vi "New Parameterized Test Case.vi"(8 "error in (no error)":errorcluster) -> (0 "error out":errorcluster)   [LabVIEW 2020]
uses:
  <vilib>/Utility/error.llb/Error Cluster From Error Code.vi
  <vilib>/ErrorRing/Error Ring.xnode
panel:
  in  "Debug?":bool
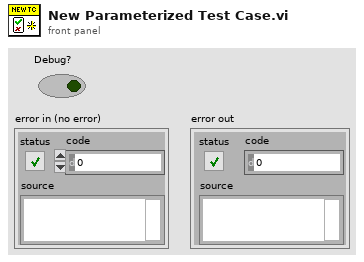
[diagram p1: front panel]
types:
  T1 = enum32{"Invalid", "Standard", "Closed", "Hidden", "Minimized", "Maximized"}
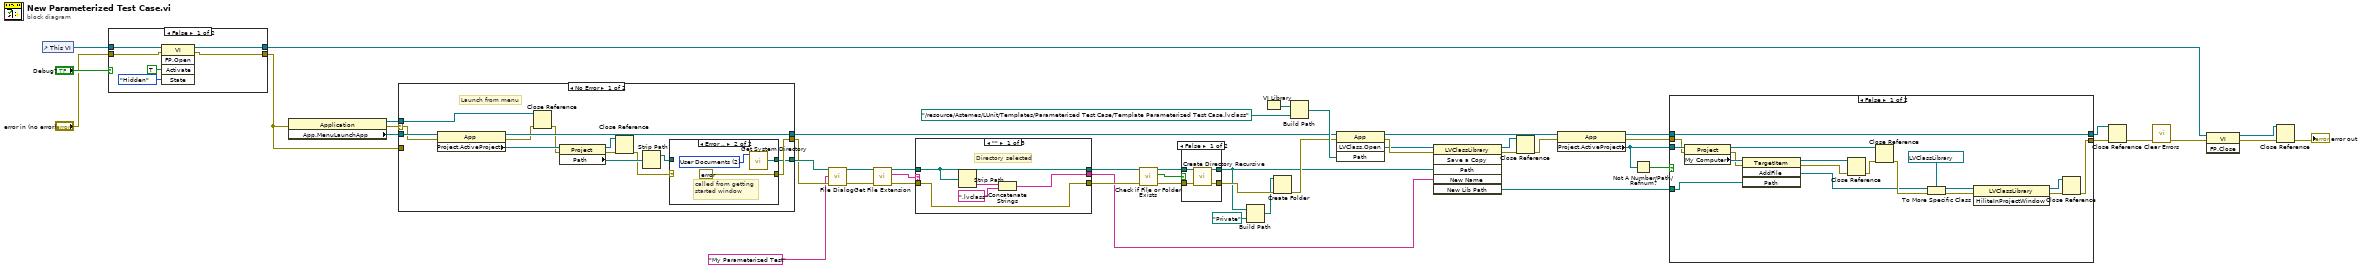
[diagram p0: block diagram]
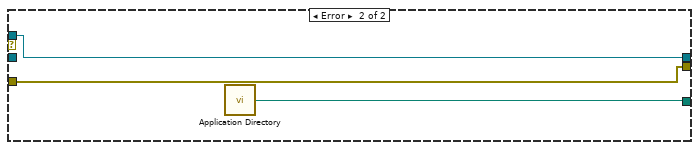
[diagram p3: hidden frame]
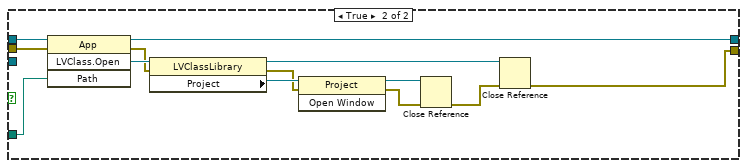
[diagram p5: hidden frame]
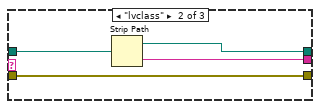
[diagram p6: hidden frame]
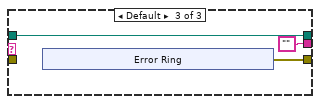
[diagram p7: hidden frame]
diagram:
  n1 = control-ref of="This VI"() -> (w21:refnum<vi>)
  n2 = case shown="False" "Debug?" {
    tunnel: w21 -> [w55 w57]
    tunnel: [w54 w57] -> w19
    tunnel: "error in (no error)" -> [w51 w56]
    tunnel: [w50 w56] -> w10
    frame False {
      n3 = invoke class="VI" method="FP.Open"(reference=w55, error in=w51, "Activate"=TRUE ("Activate?"), "State"=T1."Hidden") -> (reference out=w54:refnum<vi>, error out=w50:errorcluster)  [unwired: 1 in, 3 out]
    }
    frame True {
    }
  }
  n4 = property class="Application"(error in=w10) -> (reference out=w16:refnum<vi>, error out=w24:errorcluster, "App.MenuLaunchApp"=w49:refnum<vi>)  [unwired: 1 in]
  n5 = case shown="No Error" w24 {
    selector: w24 -> [w66 _]
    tunnel: [w69 w79] -> w12
    tunnel: w49 -> [w67 _]
    tunnel: [w60 w78] -> w8
    tunnel: w10 -> [_ w78]
    tunnel: w16 -> [w71 w79]
    tunnel: [w59 w77] -> w9
    frame No Error {
      # "Launch from menu"
      n6 = property class="App"(reference=w67, error in=w66) -> (reference out=w69:refnum<vi>, error out=w68:errorcluster, "Project.ActiveProject"=w70:refnum<vi>)
      n7 = Close Reference(reference=w71, error in (no error)=w68) -> (error out=w65:errorcluster)
      n8 = property class="Project"(reference=w70, error in=w65) -> (reference out=w63:refnum<vi>, error out=w64:errorcluster, "Path"=w62:path)
      n9 = Close Reference(reference=w63, error in (no error)=w64) -> (error out=w61:errorcluster)
      n10 = Strip Path(path=w62) -> (stripped path=w58:path)  [unwired: 1 out]
      n11 = case shown="Error .." w61 {
        selector: w61 -> [w73 _]
        tunnel: [w73 errorcluster {"status"=FALSE, "code"=0, "source"=""} ("error IO")] -> w60
        tunnel: [w72 w74] -> w59
        tunnel: w58 -> [w72 _]
        frame No Error {
        }
        frame Error {
          w75 = 2 items=["User Home"=0, "User Desktop"=1, "User Documents"=2, "User Application Data"=3, "User Preferences"=4, "User Temporary"=5, "Public Documents"=6, "Public Application Data"=7, "Public Preferences"=8, "Public Cache"=13, "System Core Libraries"=9, "System Installed Libraries"=10, "Application Files"=11, "Boot Volume Root"=12] ("system directory type")
          # "called from getting started window"
          n12 = call <vilib>:"Get System Directory.vi"("system directory type"=w75) -> ("system directory"=w74:path)  [unwired: 10 in]
        }
      }
    }
    frame Error {
      n13 = call <vilib>:"Application Directory.vi"() -> ("Application Directory"=w77:path)
    }
  }
  n14 = call "File Dialog"("start path"=w9, "default name"="My Parameterized Test", "error in"=w8) -> ("selected path"=w45:path, "error out"=w7:errorcluster)  [unwired: 9 in, 2 out]
  n15 = call <vilib>:"Get File Extension.vi"("error in (no error)"=w7, "file"=w45) -> ("error out"=w48:errorcluster, "lowercase file extension"=w47:string, "dup file"=w46:path)  [unwired: 5 in, 2 out]
  n16 = case shown="\"\"" w47 {
    tunnel: w48 -> [w80 w85 _]
    tunnel: w46 -> [w81 w88 w89]
    tunnel: [w80 w85 w91] -> w43
    tunnel: [w82 w87 "" ("name")] -> w39
    tunnel: [w81 w86 w89] -> w44
    frame "" {
      # "Directory selected"
      n17 = Strip Path(path=w81) -> (name=w84:string)  [unwired: 1 out]
      n18 = Concatenate Strings(w84, ".lvclass" ("string")) -> (w82:string)
    }
    frame "lvclass" {
      n19 = Strip Path(path=w88) -> (stripped path=w86:path, name=w87:string)
    }
    frame Default {
      n20 = xnode "Error Ring"() -> ("error out"=w91:errorcluster)
    }
  }
  n21 = call <vilib>:"Check if File or Folder Exists.vi"("error in (no error)"=w43, "path"=w44) -> ("error out"=w42:errorcluster, "file or folder exists?"=w40:bool, "dup path"=w41:path)  [unwired: 7 in]
  n22 = case shown="False" w40 {
    tunnel: w42 -> [w99 w100]
    tunnel: w41 -> [w98 w101]
    tunnel: [w97 w101] -> w3
    tunnel: [w96 w100] -> w6
    frame False {
      n23 = call <vilib>:"Create Directory Recursive.vi"("error in (no error)"=w99, "directory"=w98) -> ("error out"=w96:errorcluster, "directory copy"=w97:path)  [unwired: 3 in, 1 out]
    }
    frame True {
    }
  }
  n24 = Build Path(base path=w3, name or relative path=path "Private") -> (appended path=w1:path)
  n25 = VI Library() -> (path=w30:path)
  n26 = Create Folder(path (use dialog)=w1, error in=w6) -> (error out=w4:errorcluster)  [unwired: 1 in, 2 out]
  n27 = Build Path(base path=w30, name or relative path=path "../resource/Astemes/LUnit/Templates/Parameterized Test Case/Template Parameterized Test Case.lvclass") -> (appended path=w28:path)
  n28 = invoke class="App" method="LVClass.Open"(reference=w12, error in=w4, "Path"=w28) -> (reference out=w25:refnum<vi>, error out=w38:errorcluster, "LVClass.Open"=w17:refnum<vi>)  [unwired: 1 in, 1 out]
  n29 = invoke class="LVClassLibrary" method="Save a Copy"(reference=w17, error in=w38, "Path"=w3, "New Name"=w39) -> (reference out=w26:refnum<vi>, error out=w23:errorcluster, "New Lib Path"=w34:path)  [unwired: 2 in, 3 out]
  n30 = Close Reference(reference=w26, error in (no error)=w23) -> (error out=w22:errorcluster)
  n31 = property class="App"(reference=w25, error in=w22) -> (reference out=w33:refnum<vi>, error out=w35:errorcluster, "Project.ActiveProject"=w36:refnum<vi>)
  n32 = Not A Number/Path/Refnum?(number/path/refnum=w36) -> (NaN/Path/Refnum?=w37:bool)
  n33 = case shown="False" w37 {
    tunnel: w36 -> [w119 _]
    tunnel: w35 -> [w117 w123]
    tunnel: w34 -> [w111 w121]
    tunnel: [w106 w120] -> w31
    tunnel: w33 -> [w110 w124]
    tunnel: [w110 w122] -> w32
    frame False {
      n34 = property class="Project"(reference=w119, error in=w117) -> (reference out=w113:refnum<vi>, error out=w116:errorcluster, "My Computer"=w118:refnum<vi>)
      n35 = invoke class="TargetItem" method="AddFile"(reference=w118, error in=w116, "Path"=w111) -> (reference out=w114:refnum<vi>, error out=w115:errorcluster, "AddFile"=w102:refnum<vi>)  [unwired: 1 in, 1 out]
      n36 = Close Reference(reference=w114, error in (no error)=w115) -> (error out=w112:errorcluster)
      n37 = Close Reference(reference=w113, error in (no error)=w112) -> (error out=w109:errorcluster)
      n38 = To More Specific Class(target class=refnum<vi> refnum ("reference"), reference=w102, error in=w109) -> (specific class reference=w103:refnum<vi>, error out=w105:errorcluster)
      n39 = invoke class="LVClassLibrary" method="HiliteInProjectWindow"(reference=w103, error in=w105) -> (reference out=w107:refnum<vi>, error out=w108:errorcluster)  [unwired: 1 in, 1 out]
      n40 = Close Reference(reference=w107, error in (no error)=w108) -> (error out=w106:errorcluster)
    }
    frame True {
      n41 = invoke class="App" method="LVClass.Open"(reference=w124, error in=w123, "Path"=w121) -> (reference out=w122:refnum<vi>, error out=w131:errorcluster, "LVClass.Open"=w132:refnum<vi>)  [unwired: 1 in, 1 out]
      n42 = property class="LVClassLibrary"(reference=w132, error in=w131) -> (reference out=w130:refnum<vi>, error out=w128:errorcluster, "Project"=w129:refnum<vi>)
      n43 = invoke class="Project" method="Open Window"(reference=w129, error in=w128) -> (reference out=w127:refnum<vi>, error out=w126:errorcluster)  [unwired: 1 in, 1 out]
      n44 = Close Reference(reference=w127, error in (no error)=w126) -> (error out=w125:errorcluster)
      n45 = Close Reference(reference=w130, error in (no error)=w125) -> (error out=w120:errorcluster)
    }
  }
  n46 = Close Reference(reference=w32, error in (no error)=w31) -> (error out=w27:errorcluster)
  n47 = call <vilib>:"Clear Errors.vi"("error in (no error)"=w27) -> ("error out"=w13:errorcluster)  [unwired: 5 in, 1 out]
  n48 = invoke class="VI" method="FP.Close"(reference=w19, error in=w13) -> (reference out=w15:refnum<vi>, error out=w14:errorcluster)  [unwired: 1 in, 1 out]
  n49 = Close Reference(reference=w15, error in (no error)=w14) -> (error out=→"error out":errorcluster)
